vi "Wire Close Sessions.vi"(0 "sub vis ref":refnum<vi>[](array[refnum]), 11 "error in":errorcluster) -> (15 "error out":errorcluster)   [LabVIEW 2021, in "Converter.lvlib"]
uses:
  Converter.lvlib
  Converter Reusables/Converter Reusables.lvlib
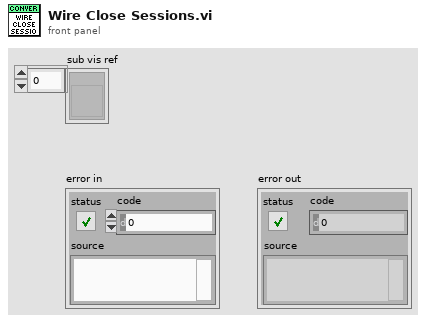
[diagram p1: front panel]
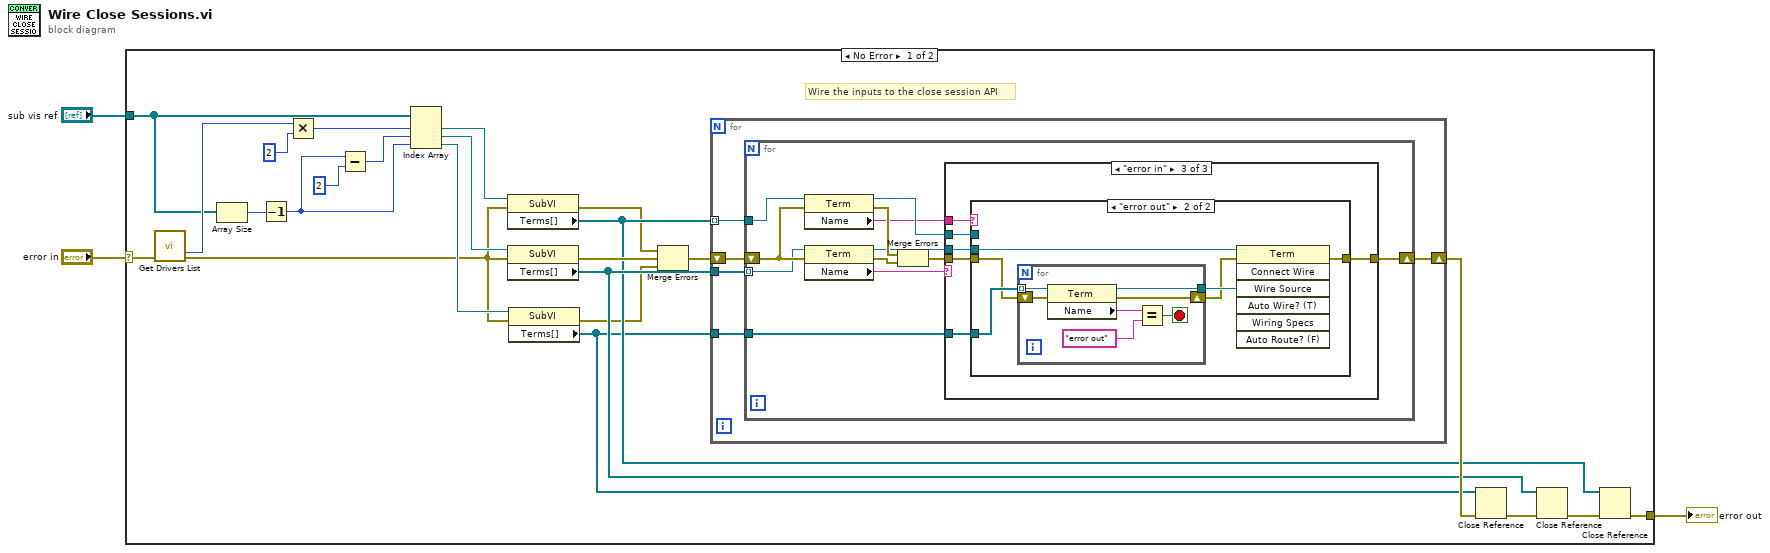
[diagram p0: block diagram]
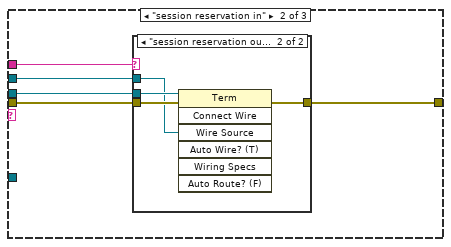
[diagram p3: hidden frame]
diagram:
  n1 = case shown="No Error" "error in" {
    selector: "error in" -> [w5 w75]
    tunnel: [w6 w75] -> w1
    tunnel: "sub vis ref" -> [w4 _]
    frame No Error {
      # "Wire the inputs to the close session API"
      n2 = call "Get Drivers List.vi"() -> ("removed duplicates size"=w8:i32)  [unwired: 10 in, 5 out]
      n3 = Array Size(array=w4) -> (size(s)=w13:i32)
      n4 = Decrement(x=w13) -> (x-1=w12:i32)
      n5 = Multiply(x=w8, y=2 ("x")) -> (x*y=w9:i32)
      n6 = Subtract(x=w12, y=2) -> (x-y=w10:i32)
      n7 = Index Array(array=w4, index #1=w9, index #2=w10, index #3=w12) -> (element #1=w21:refnum<vi>, element #2=w20:refnum<vi>, element #3=w19:refnum<vi>)
      n8 = property class="SubVI"(reference=w21, error in=w5) -> (error out=w15:errorcluster, "Terms[]"=w22:refnum<vi>[])  [unwired: 1 out]
      n9 = property class="SubVI"(reference=w20, error in=w5) -> (error out=w26:errorcluster, "Terms[]"=w23:refnum<vi>[])  [unwired: 1 out]
      n10 = property class="SubVI"(reference=w19, error in=w5) -> (error out=w14:errorcluster, "Terms[]"=w18:refnum<vi>[])  [unwired: 1 out]
      n11 = Merge Errors(w15, w26, w14) -> (w16:errorcluster)
      n12 = for {
        tunnel: w22 -> [w30] mode=indexing
        tunnel: w23 -> [w31]
        tunnel: w18 -> [w28]
        shift-right: [w27] -> w25
        shift-left: w16 -> [w29]
        n13 = for {
          tunnel: w31 -> [w34] mode=indexing
          tunnel: w30 -> [w43]
          tunnel: w28 -> [w39]
          shift-right: [w40] -> w27
          shift-left: w29 -> [w35]
          n14 = property class="Term"(reference=w43, error in=w35) -> (reference out=w41:refnum<vi>, error out=w37:errorcluster, "Name"=w32:string)
          n15 = property class="Term"(reference=w34, error in=w35) -> (reference out=w36:refnum<vi>, error out=w42:errorcluster, "Name"=w33:string)
          n16 = Merge Errors(w37, w42) -> (w38:errorcluster)
          n17 = case shown="\"error in\"" w33 {
            tunnel: w32 -> [_ w49 w55]
            tunnel: w36 -> [_ w45 w59]
            tunnel: w38 -> [w44 w48 w60]
            tunnel: [w44 w46 w57] -> w40
            tunnel: w41 -> [_ w47 w58]
            tunnel: w39 -> [_ _ w56]
            frame Default {
            }
            frame "session reservation in" {
              n18 = case shown="\"session reservation out\"" w49 {
                tunnel: w48 -> [w50 w54]
                tunnel: w45 -> [_ w52]
                tunnel: w47 -> [_ w51]
                tunnel: [w50 w53] -> w46
                frame Default {
                }
                frame "session reservation out" {
                  n19 = invoke class="Term" method="Connect Wire"(reference=w52, error in=w54, "Wire Source"=w51) -> (error out=w53:errorcluster)  [unwired: 4 in, 6 out]
                }
              }
            }
            frame "error in" {
              n20 = case shown="\"error out\"" w55 {
                tunnel: w60 -> [w61 w63]
                tunnel: w59 -> [_ w67]
                tunnel: w58 -> [_ _]
                tunnel: [w61 w62] -> w57
                tunnel: w56 -> [_ w66]
                frame Default {
                }
                frame "error out" {
                  n21 = for {
                    tunnel: w66 -> [w74] mode=indexing
                    tunnel: [w71] -> w65
                    shift-right: [w73] -> w64
                    shift-left: w63 -> [w72]
                    stop <- w70 stop-if-true
                    n22 = property class="Term"(reference=w74, error in=w72) -> (reference out=w71:refnum<vi>, error out=w73:errorcluster, "Name"=w69:string)
                    n23 = Equal?(x=w69, y="error out") -> (x = y?=w70:bool)
                  }
                  n24 = invoke class="Term" method="Connect Wire"(reference=w67, error in=w64, "Wire Source"=w65) -> (error out=w62:errorcluster)  [unwired: 4 in, 6 out]
                }
              }
            }
          }
        }
      }
      n25 = Close Reference(reference=w18, error in (no error)=w25) -> (error out=w17:errorcluster)
      n26 = Close Reference(reference=w23, error in (no error)=w17) -> (error out=w24:errorcluster)
      n27 = Close Reference(reference=w22, error in (no error)=w24) -> (error out=w6:errorcluster)
    }
    frame Error {
    }
  }
  "error out" <- w1
